vi "Create_directory_path.vi"(2 "error in (no error)":errorcluster, 3 "Path name":path) -> (0 "error out":errorcluster, 1 "Path name Out":path)   [LabVIEW 2013]
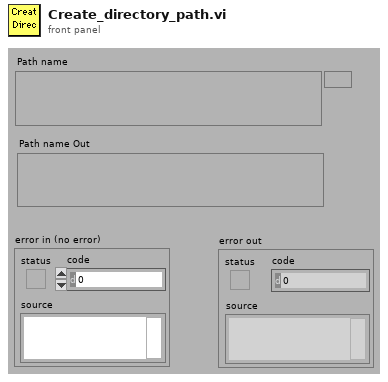
[diagram p1: front panel]
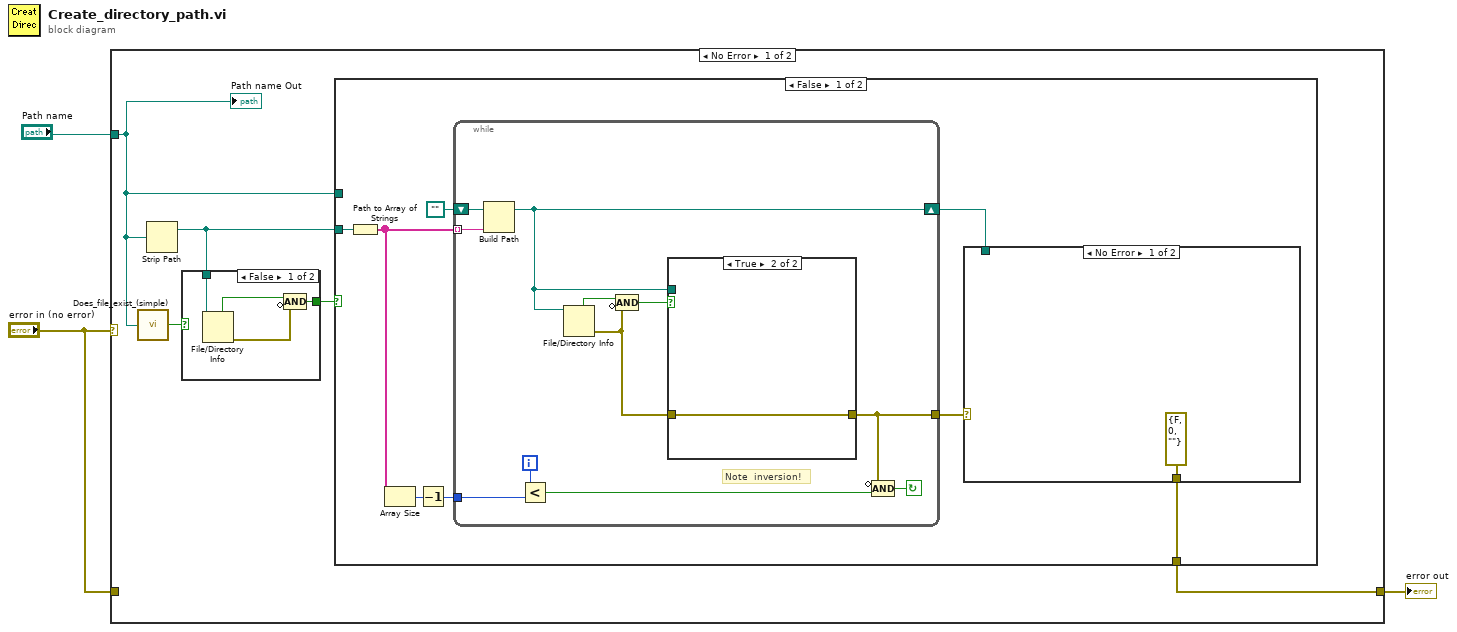
[diagram p0: block diagram]
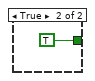
[diagram p2: hidden frame]
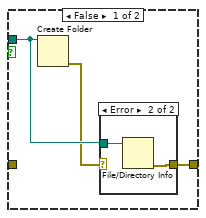
[diagram p3: hidden frame]
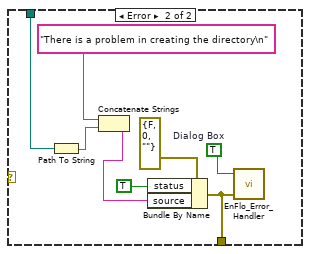
[diagram p5: hidden frame]
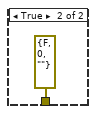
[diagram p6: hidden frame]
diagram:
  n1 = case shown="No Error" "error in (no error)" {
    tunnel: [w5 w50] -> w3
    tunnel: "error in (no error)" -> [_ w50]
    tunnel: "Path name" -> [w4 _]
    frame No Error {
      n2 = call "Does_file_exist_(simple).vi"("Pathname"=w4) -> ("exists?"=w6:bool)
      n3 = Strip Path(path=w4) -> (stripped path=w7:path)  [unwired: 1 out]
      n4 = case shown="False" w6 {
        tunnel: [w12 TRUE] -> w8
        tunnel: w7 -> [w10 _]
        frame False {
          n5 = File/Directory Info(path=w10) -> (directory=w11:bool, error out=w9:errorcluster)  [unwired: 1 in, 5 out]
          n6 = Compound Arithmetic op=AND(w11, invert w9) -> (w12:bool)
        }
        frame True {
        }
      }
      n7 = case shown="False" w8 {
        tunnel: w4 -> [_ _]
        tunnel: w7 -> [w16 _]
        tunnel: [w14 errorcluster {"status"=FALSE, "code"=0, "source"=""} ("error in (no error)")] -> w5
        frame False {
          n8 = Path to Array of Strings(0:w16) -> (2:w20:string[])  [unwired: 1 out]
          n9 = Array Size(array=w20) -> (size(s)=w15:i32)
          n10 = Decrement(x=w15) -> (x-1=w17:i32)
          n11 = while {
            tunnel: [w26] -> w19
            tunnel: w17 -> [w29]
            shift-left: path "" ("appended path") -> [w32]
            shift-right: [w25] -> w18
            tunnel: w20 -> [w31] mode=indexing
            i -> [w30]
            stop <- w27 continue-if-true
            # "Note  inversion!"
            n12 = Build Path(base path=w32, name or relative path=w31) -> (appended path=w25:path)
            n13 = Less?(x=w30, y=w29) -> (x < y?=w28:bool)
            n14 = File/Directory Info(path=w25) -> (directory=w24:bool, error out=w22:errorcluster)  [unwired: 1 in, 5 out]
            n15 = Compound Arithmetic op=AND(w24, invert w22) -> (w23:bool)
            n16 = case shown="True" w23 {
              tunnel: w25 -> [w35 _]
              tunnel: [w33 w39] -> w26
              tunnel: w22 -> [_ w39]
              frame False {
                n17 = Create Folder(path (use dialog)=w35) -> (error out=w34:errorcluster)  [unwired: 1 in, 3 out]
                n18 = case shown="Error" w34 {
                  selector: w34 -> [w36 _]
                  tunnel: w35 -> [_ w38]
                  tunnel: [w36 w37] -> w33
                  frame No Error {
                  }
                  frame Error {
                    n19 = File/Directory Info(path=w38) -> (error out=w37:errorcluster)  [unwired: 1 in, 6 out]
                  }
                }
              }
              frame True {
              }
            }
            n20 = Compound Arithmetic op=AND(invert w26, w28) -> (w27:bool)
          }
          n21 = case shown="No Error" w19 {
            tunnel: w18 -> [_ w48]
            tunnel: [errorcluster {"status"=FALSE, "code"=0, "source"=""} ("error in (no error)") w41] -> w14
            frame No Error {
            }
            frame Error {
              w44 = TRUE  # Dialog Box
              n22 = Path To String(path=w48) -> (string=w46:string)
              n23 = Concatenate Strings("There is a problem in creating the directory\n", w46) -> (w42:string)
              n24 = Bundle By Name(cluster=errorcluster {"status"=FALSE, "code"=0, "source"=""} ("error in (no error)"), "status"=TRUE ("Bundle Element"), "source"=w42) -> (w41:errorcluster)
              n25 = call "EnFlo_Error_Handler.vi"("error in (no error)"=w41, "Dialog Box (T)"=w44) -> ()  [unwired: 1 in, 3 out]
            }
          }
        }
        frame True {
        }
      }
      "Path name Out" <- w4
    }
    frame Error {
    }
  }
  "error out" <- w3
